vi "ShooterWrapper.vi"(6 "Action":T1, 7 "error in":errorcluster) -> (0 "error out":errorcluster)   [LabVIEW 2013]
doc: "CheckedShooter is used during a normal shooting sequence (either during one-ball autonomous or teleop). It controls the shooting pneumatics (through Shooter.vi), but it ALSO checks preconditions: the collector arm, the clappers, and the roller. It has the following actions:\n-Init: take two double solenoid references and store them (one for the clapper, one for the roller). Take two single solenoid references and use them to initialize Shooter.vi (one for the firing cylinder, one for the kicker).\n-Shoot:\n +Check if the collector is up (hitting the top limit switch). (Only if CheckLimitSwitch is true.)\n +Actuate the roller to out.\n +Actuate the clapper to middle.\n +Shoot (using Shooter.vi). Wait1, Wait2, and Wait3 correspond to the waits used by Shooter.vi."
uses:
  ShooterWrapperAction.ctl
  ShooterAction.ctl
  DoubleSolenoidAction.ctl
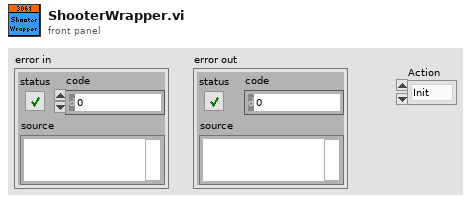
[diagram p1: front panel]
types:
  T1 = typedef "ShooterWrapperAction.ctl" = enum16{"Init", "CollectorDown", "CollectorUp"}
  T2 = typedef "ShooterAction.ctl" = enum16{"Init", "Shoot"}
  T3 = typedef "DoubleSolenoidAction.ctl" = enum16{"Init", "Middle", "In", "Out"}
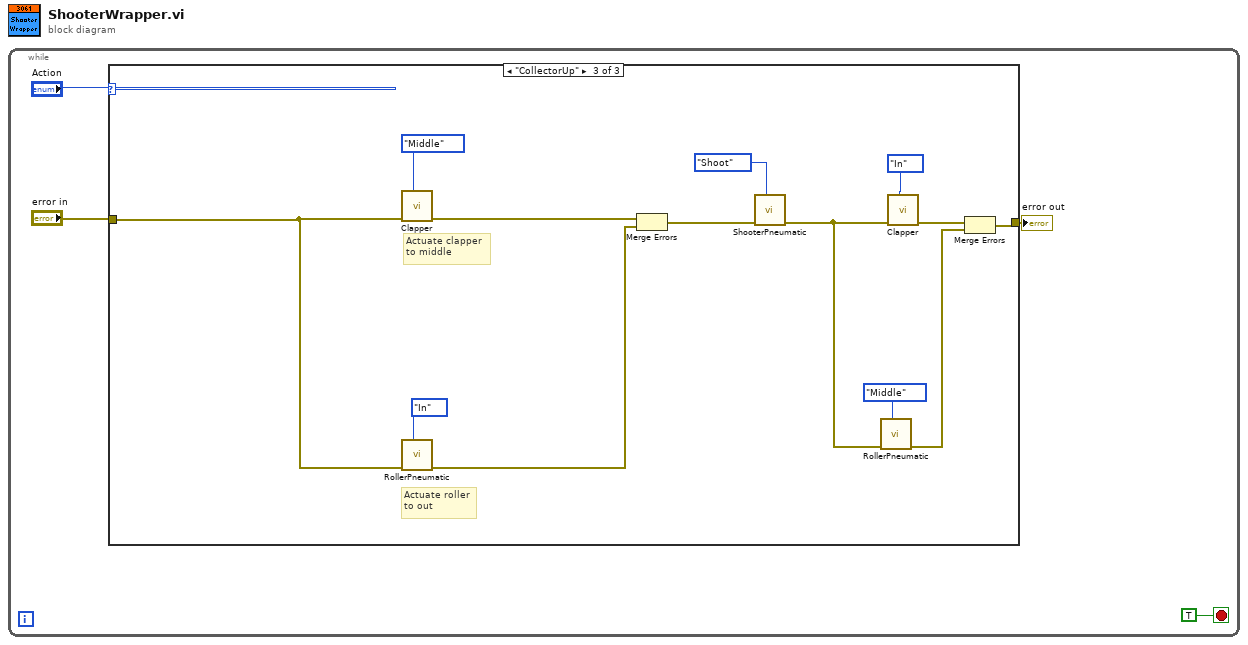
[diagram p0: block diagram]
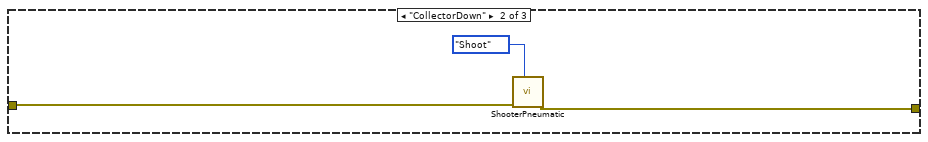
[diagram p3: hidden frame]
diagram:
  n1 = while {
    stop <- TRUE stop-if-true
    n2 = case shown="\"CollectorUp\"" "Action" {
      tunnel: "error in" -> [w5 w6 w15]
      tunnel: [w5 w7 w11] -> w1
      frame "Init", Default {
      }
      frame "CollectorDown" {
        n3 = call "ShooterPneumatic.vi"("Action"=ShooterAction."Shoot", "error in"=w6) -> ("error out"=w7:errorcluster)  [unwired: 9 in]
      }
      frame "CollectorUp" {
        # "Actuate clapper\nto middle"
        # "Actuate roller\nto out"
        n4 = call "Clapper.vi"("State"=DoubleSolenoidAction."Middle", "Error in"=w15) -> ("Error out"=w17:errorcluster)  [unwired: 9 in]
        n5 = call "RollerPneumatic.vi"("State"=DoubleSolenoidAction."In", "Error in"=w15) -> ("Error out"=w16:errorcluster)  [unwired: 9 in]
        n6 = Merge Errors(w17, w16) -> (w18:errorcluster)
        n7 = call "ShooterPneumatic.vi"("Action"=ShooterAction."Shoot", "error in"=w18) -> ("error out"=w12:errorcluster)  [unwired: 9 in]
        n8 = call "RollerPneumatic.vi"("State"=DoubleSolenoidAction."Middle", "Error in"=w12) -> ("Error out"=w9:errorcluster)  [unwired: 9 in]
        n9 = call "Clapper.vi"("State"=DoubleSolenoidAction."In", "Error in"=w12) -> ("Error out"=w10:errorcluster)  [unwired: 9 in]
        n10 = Merge Errors(w10, w9) -> (w11:errorcluster)
      }
    }
    "error out" <- w1
  }
